vi "Wait For Bytes.vi"(8 "error in (no error)":errorcluster, 10 "Bytes To Read (0)":u32, 11 "VISA resource name":refnum<visa-resource-name>) -> (0 "error out":errorcluster, 3 "VISA resource name out":refnum<visa-resource-name>)   [LabVIEW 2012, in "MicroStrain 3DM-GXx.lvlib"]
doc: "Wait for the specified number of bytes to be available in the VISA buffer."
uses:
  <instrlib>/MicroStrain 3DM-GXx/MicroStrain 3DM-GXx.lvlib
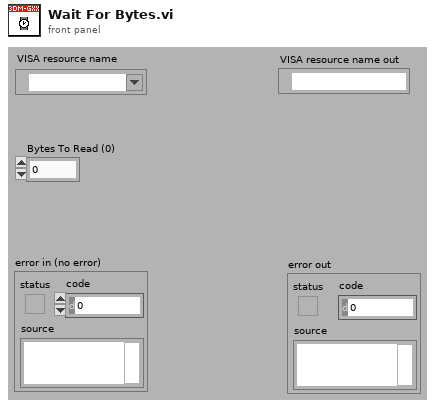
[diagram p1: front panel]
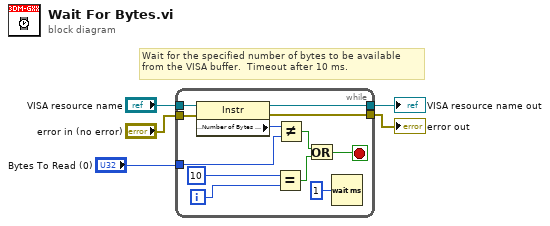
[diagram p0: block diagram]
diagram:
  # "Wait for the specified number of bytes to be available\nfrom the VISA buffer.  Timeout after 10 ms."
  n1 = while {
    tunnel: "Bytes To Read (0)" -> [w16]
    tunnel: [w15] -> w3
    tunnel: [w14] -> w2
    tunnel: "VISA resource name" -> [w7]
    tunnel: "error in (no error)" -> [w6]
    i -> [w11]
    stop <- w8 stop-if-true
    n2 = property class="Instr"(reference=w7, error in=w6) -> (reference out=w15:refnum<visa-resource-name>, error out=w14:errorcluster, "Serial Settings:Number of Bytes at Serial Port"=w17:u32)
    n3 = Equal?(x=10, y=w11) -> (x = y?=w9:bool)
    n4 = Not Equal?(x=w17, y=w16) -> (x != y?=w12:bool)
    n5 = Or(x=w12, y=w9) -> (x .or. y?=w8:bool)
    n6 = Wait (ms)(milliseconds to wait=u32 1) -> ()  [unwired: 1 out]
  }
  "VISA resource name out" <- w3
  "error out" <- w2
